vi "gestoscidwie_subIV.vi"(10 "time":dbl, 11 "wykres":waveform(dbl)) -> (1 "wykres 3":waveform(dbl), 2 "wykres 2":waveform(dbl), 3 "as":cdb[](array[numeric]), 4 "df":dbl, 5 "n2":dbl)   [LabVIEW 2025]
uses:
  <vilib>/Analysis/2dsp.llb/Real FFT.vi
  <vilib>/Analysis/NI_AALPro.lvlib
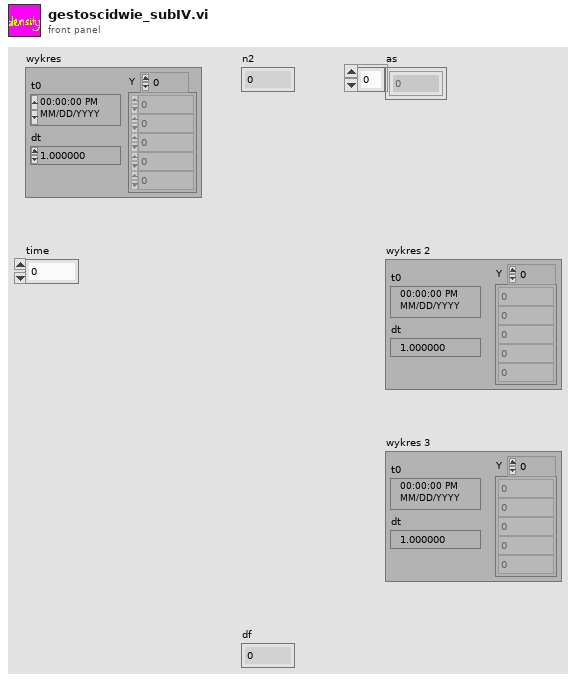
[diagram p1: front panel]
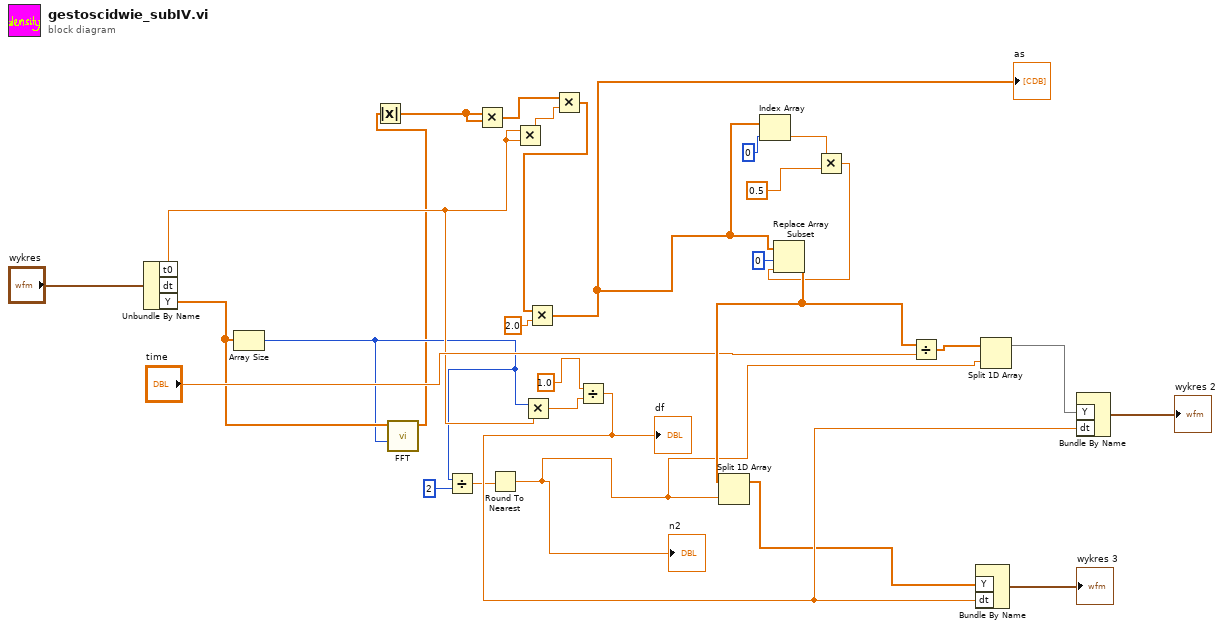
[diagram p0: block diagram]
diagram:
  n1 = Unbundle By Name("wykres") -> ("dt"=w16:dbl, "Y"=w14:dbl[])  [unwired: 1 out]
  n2 = Array Size(array=w14) -> (size(s)=w10:i32)
  n3 = call-poly <vilib>:"FFT.vi"("FFT size"=w10, "X"=w14) -> ("FFT {X}"=w7:cdb[])  [unwired: 8 in, 1 out]
  n4 = Absolute Value(x=w7) -> (abs(x)=w15:dbl[])
  n5 = Divide(x=w10, y=2) -> (x/y=w8:dbl)
  n6 = Multiply(x=w15, y=w15) -> (x*y=w17:dbl[])
  n7 = Round To Nearest(number=w8) -> (nearest integer value=w1:dbl)
  "n2" <- w1
  n8 = Multiply(x=w16, y=w16) -> (x*y=w18:dbl)
  n9 = Multiply(x=w10, y=w16) -> (x*y=w11:dbl)
  n10 = Multiply(x=w17, y=w18) -> (x*y=w19:dbl[])
  n11 = Multiply(x=w19, y=2.0) -> (x*y=w26:dbl[])
  "as" <- w26
  n12 = Divide(x=1.0, y=w11) -> (x/y=w28:dbl)
  "df" <- w28
  n13 = Index Array(array=w26, index=0) -> (element=w23:dbl)
  n14 = Multiply(x=w23, y=0.5) -> (x*y=w22:dbl)
  n15 = Replace Array Subset(array=w26, new element=w22, index=0) -> (w27:dbl[])
  n16 = Split 1D Array(array=w27, index=w1) -> (first subarray=w5:dbl[])  [unwired: 1 out]
  n17 = Divide(x=w27, y="time") -> (x/y=w3:dbl[])
  n18 = Bundle By Name("Y"=w5, "dt"=w28) -> (→"wykres 3":waveform(dbl))  [unwired: 1 in]
  n19 = Split 1D Array(array=w3, index=w1) -> (first subarray=w2:dbl[])  [unwired: 1 out]
  n20 = Bundle By Name("Y"=w2, "dt"=w28) -> (→"wykres 2":waveform(dbl))  [unwired: 1 in]
